vi "Change_Windows_IPconfig.vi"() -> ()   [LabVIEW 2016]
panel:
  out "standard output":string
  in  "Static      DHCP":bool
  in  "metric":string
  in  "default gateway":string
  in  "mask":string="255.255.255.0"
  in  "IP address":string="192.168.0.100"
  in  "connection name":string="Local Area Connection 2"
  out "error out":errorcluster
  in  "error in (no error)":errorcluster
  # "Optional Parameters"
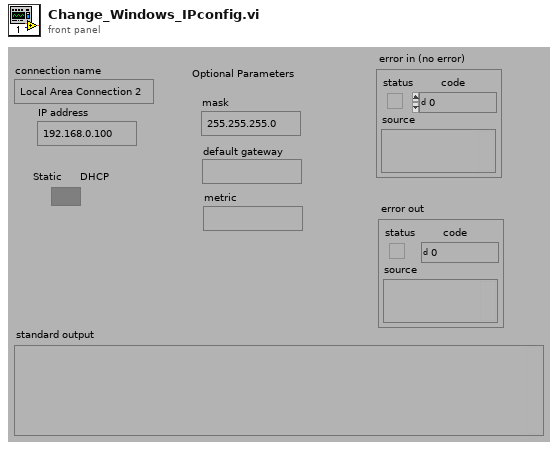
[diagram p1: front panel]
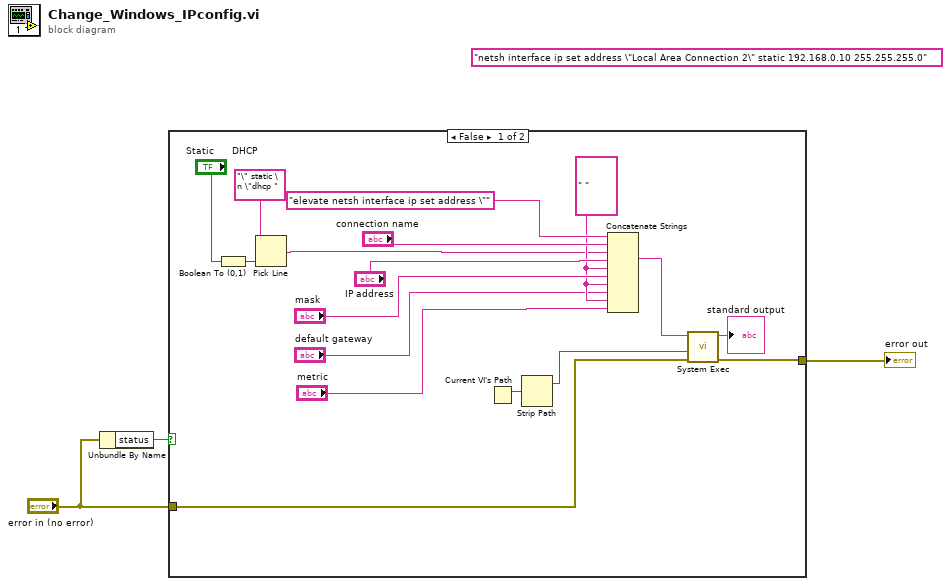
[diagram p0: block diagram]
diagram:
  (unwired) "netsh interface ip set address \"Local Area Connection 2\" static 192.168.0.10 255.255.255.0"
  n1 = Unbundle By Name("error in (no error)") -> ("status"=w1:bool)
  n2 = case shown="False" w1 {
    tunnel: "error in (no error)" -> [w20 w21]
    tunnel: [w19 w21] -> w3
    frame False {
      w14 = " " ("string")
      n3 = Boolean To (0,1)(Boolean="Static      DHCP") -> (0, 1=w8:i16)
      n4 = Pick Line(multi-line string="\" static \n \"dhcp ", line index=w8) -> (output string=w10:string)  [unwired: 1 in]
      n5 = Current VI's Path() -> (path=w5:path)
      n6 = Strip Path(path=w5) -> (stripped path=w4:path)  [unwired: 1 out]
      n7 = Concatenate Strings("elevate netsh interface ip set address \"", "connection name", w10, "IP address", w14, "mask", w14, "default gateway", w14, "metric") -> (w11:string)
      n8 = call <vilib>:"System Exec.vi"("error in (no error)"=w20, "working directory"=w4, "command line"=w11) -> ("error out"=w19:errorcluster, "standard output"=→"standard output":string)  [unwired: 5 in, 2 out]
    }
    frame True {
    }
  }
  "error out" <- w3
